vi "Read Discrete Inputs.vi"(8 "error in (no error)":errorcluster, 9 "number of discrete inputs":u16, 10 "starting address":u16, 11 "Modbus master in":refnum<class "Modbus Master.lvclass">) -> (0 "error out":errorcluster, 2 "discrete input values":bool[](array[boolean]), 3 "Modbus master out":refnum<class "Modbus Master.lvclass">)   [LabVIEW 2015, in "Modbus Master.lvclass"]
doc: "Reads values from contiguous discrete inputs. The maximum number of discrete inputs this VI can read is 2,000."
uses:
  <vilib>/Modbus/master/Modbus Master.lvclass
  <vilib>/Modbus/subvis/Modbus API/Modbus API.lvclass/Modbus API.ctl
  <vilib>/Modbus/master/Modbus Master.lvclass/Modbus Master.ctl
  <vilib>/Modbus/subvis/Protocol/Interfaces/Network Master/Network Master.lvclass
  <vilib>/Modbus/subvis/Transmission Data Unit (ADU)/Transmission Data Unit/Transmission Data Unit.lvclass
  <vilib>/Modbus/subvis/Modbus API/Modbus API.lvclass
  <vilib>/Modbus/subvis/Data and Functions/Master Function Definition/Master Function Definition.lvlib
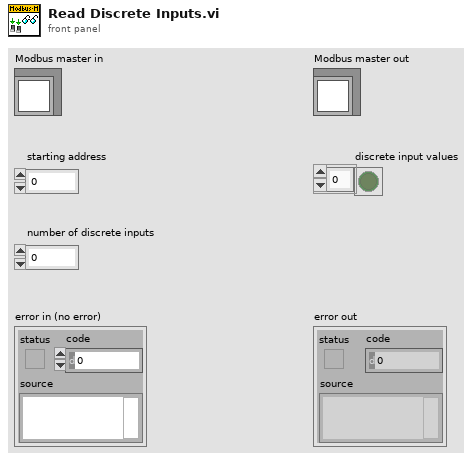
[diagram p1: front panel]
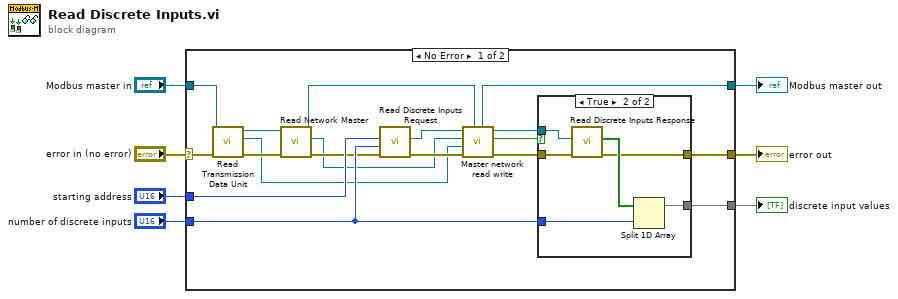
[diagram p0: block diagram]
diagram:
  n1 = case shown="No Error" "error in (no error)" {
    selector: "error in (no error)" -> [w9 w33]
    tunnel: "Modbus master in" -> [w8 w34]
    tunnel: [w17 w34] -> w6
    tunnel: [w18 w33] -> w5
    tunnel: [w23 _] -> w3
    tunnel: "number of discrete inputs" -> [w22 _]
    tunnel: "starting address" -> [w24 _]
    frame No Error {
      n2 = call <vilib>:"Read Transmission Data Unit.vi"("error in (no error)"=w9, "Modbus instance in"=w8) -> ("error out"=w15:errorcluster, "transmission data unit"=w12:refnum<class "Transmission Data Unit.lvclass">, "Modbus instance out"=w16:refnum<class "Modbus Master.lvclass">)  [unwired: 7 in]
      n3 = call <vilib>:"Read Network Master.vi"("error in (no error)"=w15, "Modbus master in"=w16) -> ("error out"=w14:errorcluster, "network master"=w11:refnum<class "Network Master.lvclass">, "Modbus master out"=w13:refnum<class "Modbus Master.lvclass">)  [unwired: 7 in]
      n4 = call <vilib>:"Read Discrete Inputs Request.vi"("error in (no error)"=w14, "number of inputs"=w22, "starting address"=w24) -> ("error out"=w25:errorcluster, "Modbus data unit out"=w20:refnum<class "Modbus Data Unit (PDU).lvclass">)  [unwired: 7 in]
      n5 = call <vilib>:"Master network read write.vi"("Modbus master in"=w13, "error in (no error)"=w25, "transmission data unit in"=w12, "network master in"=w11, "Modbus data unit in"=w20) -> ("error out"=w21:errorcluster, "PDU valid?"=w10:bool, "Modbus data unit out"=w19:refnum<class "Modbus Data Unit (PDU).lvclass">, "Modbus master out"=w17:refnum<class "Modbus Master.lvclass">)  [unwired: 3 in]
      n6 = case shown="True" w10 {
        tunnel: [_ w31] -> w23
        tunnel: w22 -> [_ w30]
        tunnel: w21 -> [w26 w29]
        tunnel: w19 -> [_ w28]
        tunnel: [w26 w27] -> w18
        frame False {
        }
        frame True {
          n7 = call <vilib>:"Read Discrete Inputs Response.vi"("error in (no error)"=w29, "Modbus data unit in"=w28) -> ("error out"=w27:errorcluster, "data"=w32:bool[])  [unwired: 8 in]
          n8 = Split 1D Array(array=w32, index=w30) -> (first subarray=w31:bool[])  [unwired: 1 out]
        }
      }
    }
    frame Error {
    }
  }
  "error out" <- w5
  "Modbus master out" <- w6
  "discrete input values" <- w3
